vi "Reserved Type.vi"(8 "error in (no error)":errorcluster, 10 "Text":string, 11 "ProtoParser in":refnum<class "ProtoParser.lvclass">) -> (0 "error out":errorcluster, 1 "Values":string[](array[string]), 2 "Reserved Type":T1, 3 "ProtoParser out":refnum<class "ProtoParser.lvclass">)   [LabVIEW 2020, in "LV-Protoc.lvlib" / "ProtoParser.lvclass"]
uses:
  ProtoParser.lvclass
  Reserved Type.ctl
  LV-Protoc.lvlib
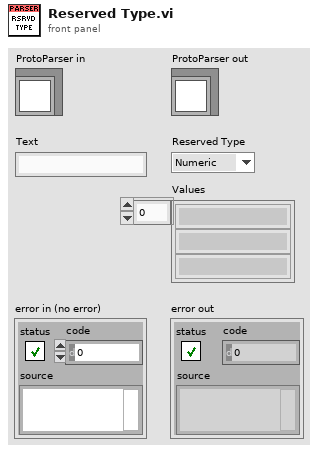
[diagram p1: front panel]
types:
  T1 = typedef "LV-Protoc.lvlib/Reserved Type.ctl" = enum16{"Numeric", "Name"}
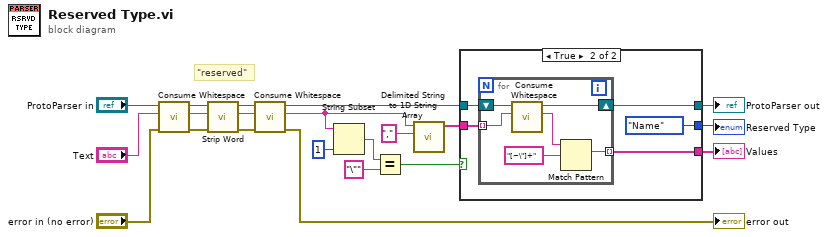
[diagram p0: block diagram]
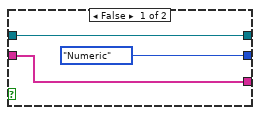
[diagram p2: hidden frame]
diagram:
  # "\"reserved\""
  n1 = call "Consume Whitespace.vi"("error in (no error)"="error in (no error)", "String"="Text", "ProtoParser in"="ProtoParser in") -> ("error out"=w3:errorcluster, "Remaining"=w18:string, "ProtoParser out"=w19:refnum<class "ProtoParser.lvclass">)  [unwired: 6 in]
  n2 = call "Strip Word.vi"("error in (no error)"=w3, "String"=w18, "ProtoParser in"=w19) -> ("error out"=w2:errorcluster, "Remaining"=w16:string, "ProtoParser out"=w17:refnum<class "ProtoParser.lvclass">)  [unwired: 5 in, 1 out]
  n3 = call "Consume Whitespace.vi"("error in (no error)"=w2, "String"=w16, "ProtoParser in"=w17) -> ("error out"=→"error out":errorcluster, "Remaining"=w7:string, "ProtoParser out"=w11:refnum<class "ProtoParser.lvclass">)  [unwired: 6 in]
  n4 = String Subset(string=w7, length (rest)=1 ("length (rest)")) -> (substring=w14:string)  [unwired: 1 in]
  n5 = Equal?(x=w14, y="\"") -> (x = y?=w12:bool)
  n6 = call <vilib>:"Delimited String to 1D String Array.vi"("delimiter"=",", "delimited string"=w7) -> ("string array"=w6:string[])  [unwired: 9 in]
  n7 = case shown="True" w12 {
    tunnel: w11 -> [w23 w26]
    tunnel: [w24 w29] -> w10
    tunnel: [w23 w25] -> w9
    tunnel: w6 -> [w24 w28]
    tunnel: [Reserved_Type."Numeric" ("Reserved Type") Reserved_Type."Name" ("Reserved Type")] -> w5
    frame False {
    }
    frame True {
      n8 = for {
        tunnel: w28 -> [w32] mode=indexing
        tunnel: [w34] -> w29 mode=indexing
        shift-right: [w30] -> w25
        shift-left: w26 -> [w33]
        n9 = call "Consume Whitespace.vi"("String"=w32, "ProtoParser in"=w33) -> ("Remaining"=w31:string, "ProtoParser out"=w30:refnum<class "ProtoParser.lvclass">)  [unwired: 7 in, 1 out]
        n10 = Match Pattern(string=w31, regular expression="[~\"]+") -> (match substring=w34:string)  [unwired: 1 in, 3 out]
      }
    }
  }
  "ProtoParser out" <- w9
  "Values" <- w10
  "Reserved Type" <- w5
